vi "Seleção das amostras mais recentes.vi"(1 "Número de amostras no gráfico":i32=2000, 2 "Vetor de entrada":dbl[](array[numeric])) -> (0 "Amostras do gráfico":dbl[](array[numeric]))   [LabVIEW 2018]
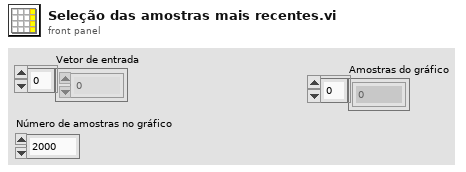
[diagram p1: front panel]
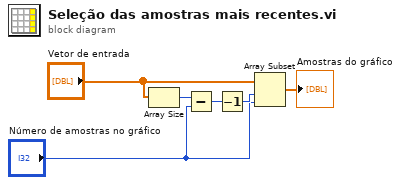
[diagram p0: block diagram]
diagram:
  n1 = Array Size(array="Vetor de entrada") -> (size(s)=w6:i32)
  n2 = Subtract(x=w6, y="Número de amostras no gráfico") -> (x-y=w5:i32)
  n3 = Decrement(x=w5) -> (x-1=w4:i32)
  n4 = Array Subset(array="Vetor de entrada", index=w4, length="Número de amostras no gráfico") -> (→"Amostras do gráfico":dbl[])
